vi "NtfyLvFpga_SUB_SettingPanel.vi"(8 "Prohibit time":T1, 10 "SendTo":T2, 11 "SMTP Setting":T3={"smtp server"="", "From"="", "port number"=25, "chk smtp auth"=FALSE, "userID"="", "password"="", "chk ssl"=FALSE}) -> (0 "Prohibit time out":T1, 1 "OK?":bool, 2 "SendTo out":T2, 3 "SMTP Setting out":T3={"smtp server"="", "From"="", "port number"=25, "chk smtp auth"=FALSE, "userID"="", "password"="", "chk ssl"=FALSE})   [LabVIEW 2013]
uses:
  <vilib>/Utility/miscctls.llb/LVPointTypeDef.ctl
panel:
  in  "Chk Prohibition":bool
  in  "End hour":u8=6 caption=":00" max=23
  in  "Start hour":u8=23 caption=":00 to" max=23
  in  "from":string caption="from address"
  in  "chk ssl":bool
  in  "chk smtp auth":bool=TRUE
  in  "password":string
  in  "userID":string
  in  "port number":i32=25
  in  "smtp server":string
  in  "To 3":string caption="To: 3"
  in  "chk To 3":bool
  in  "To 2":string="@ezweb.ne.jp" caption="To: 2"
  in  "chk To 2":bool
  in  "To 1":string caption="To: 1 (必須)"
  in  "chk To 1":bool=TRUE
  in  "Btn Test":bool
  in  "Btn Cancel":bool
  in  "Btn OK":bool
  # "Setting"
  # "SMTP Server and Account"
  # "メールサーバ"
  # "送信者メールアドレス"
  # "Notify Mail Send To:"
  # "有効"
  # "Prohibition time of mail send"
  # "の時間帯はメール送信しない。蓄積して後でまとめて送信。"
  # "同じ時刻を指定した場合は無視されます。"
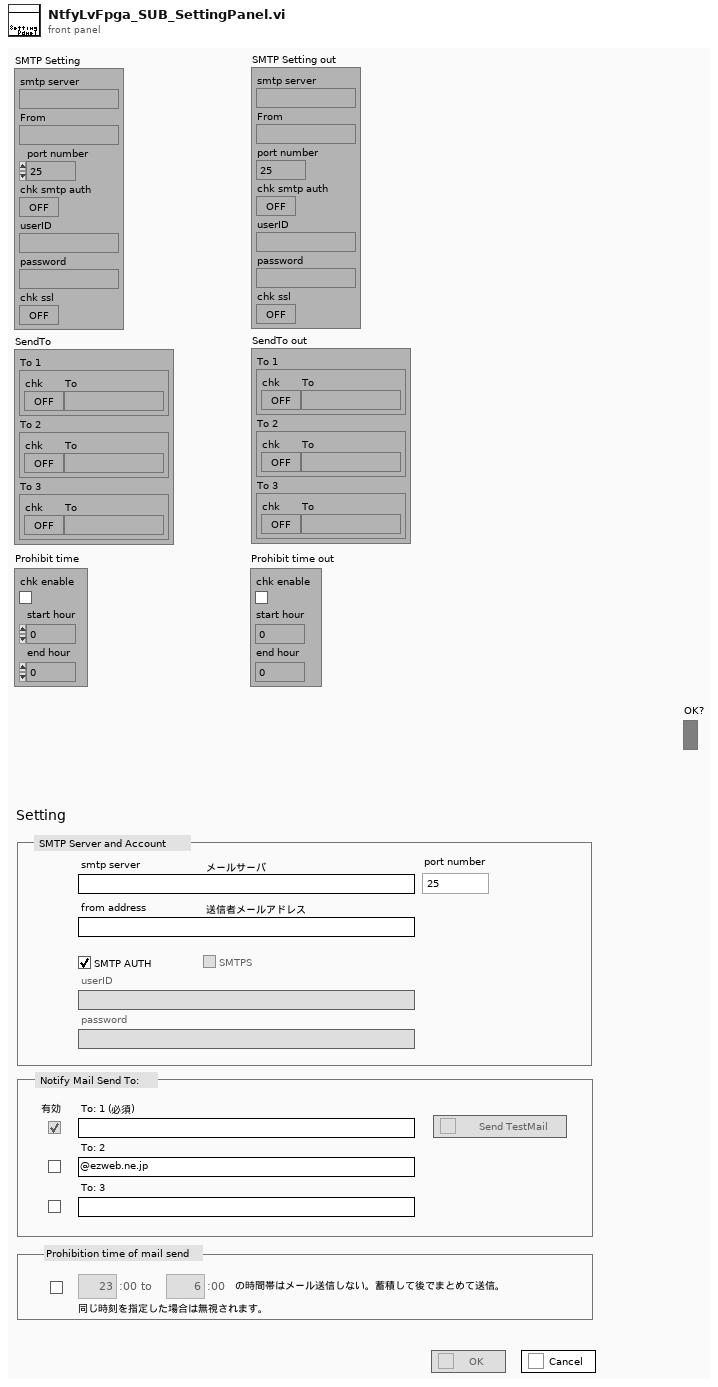
[diagram p1: front panel]
types:
  T1 = cluster{"chk enable":bool, "start hour":u8, "end hour":u8}
  T2 = cluster{"To 1":cluster{"chk":bool, "To":string}, "To 2":cluster{"chk":bool, "To":string}, "To 3":cluster{"chk":bool, "To":string}}
  T3 = cluster{"smtp server":string, "From":string, "port number":i32, "chk smtp auth":bool, "userID":string, "password":string, "chk ssl":bool}
  T4 = typedef "LVPointTypeDef.ctl" = cluster{"Horizontal":i16, "Vertical":i16}
  T5 = enum8{"Enabled", "Disabled", "Disabled and Grayed Out"}
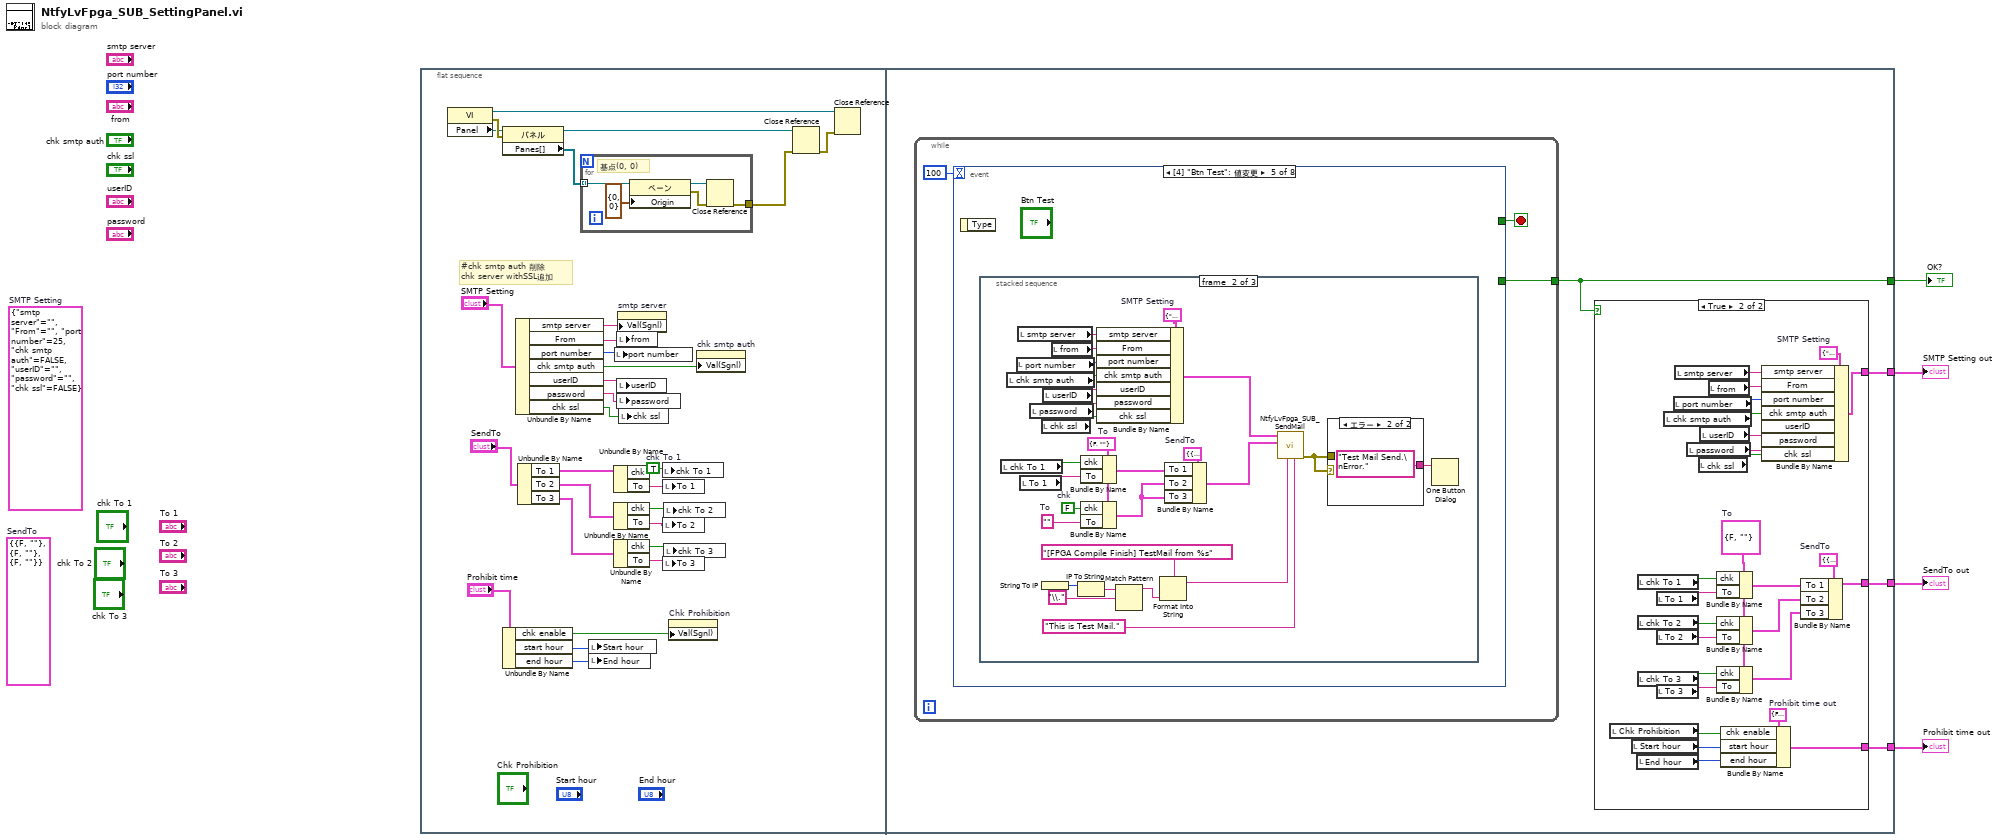
[diagram p0: block diagram]
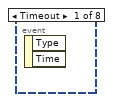
[diagram p3: hidden frame]
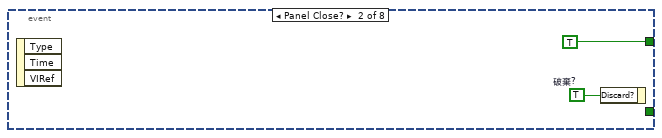
[diagram p4: hidden frame]
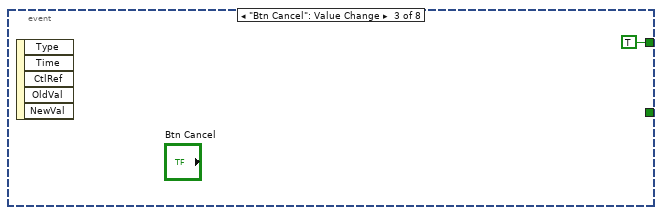
[diagram p5: hidden frame]
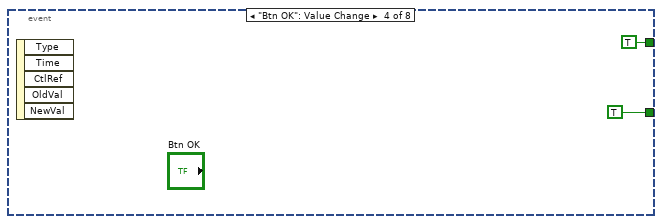
[diagram p6: hidden frame]
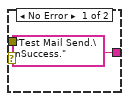
[diagram p8: hidden frame]
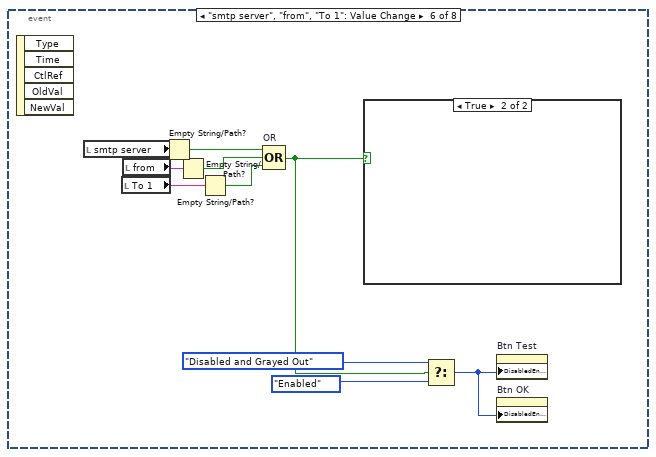
[diagram p10: hidden frame]
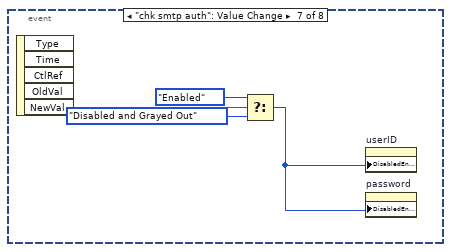
[diagram p12: hidden frame]
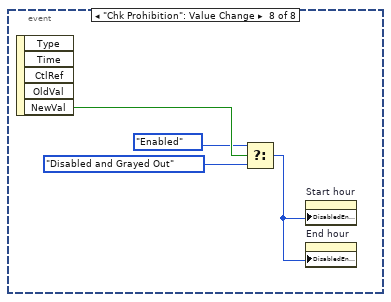
[diagram p13: hidden frame]
diagram:
  (unwired) T2 {"To 1"={"chk"=FALSE, "To"=""}, "To 2"={"chk"=FALSE, "To"=""}, "To 3"={"chk"=FALSE, "To"=""}}  # SendTo
  (unwired) T3 {"smtp server"="", "From"="", "port number"=25, "chk smtp auth"=FALSE, "userID"="", "password"="", "chk ssl"=FALSE}  # SMTP Setting
  n1 = flat-sequence {
    tunnel: [w42] -> w4
    tunnel: [w41] -> w3
    tunnel: [w40] -> w2
    tunnel: [w39] -> w1
    frame #0 {
      w11 = TRUE  # chk To 1
      # "#chk smtp auth 削除\nchk server withSSL追加"
      n2 = property class="VI"() -> (reference out=w30:refnum<vi>, error out=w33:errorcluster, "Panel"=w27:refnum<vi>)  [unwired: 2 in]
      n3 = Unbundle By Name("Prohibit time") -> ("chk enable"=w7:bool, "start hour"=w6:u8, "end hour"=w5:u8)
      n4 = property on="プロパティノード" class="パネル"(reference=w27, error in=w33) -> (reference out=w29:refnum<vi>, "Panes[]"=w28:refnum<vi>[])  [unwired: 1 out]
      n5 = Unbundle By Name("SMTP Setting") -> ("smtp server"=w10:string, "From"=w25:string, "port number"=w24:i32, "chk smtp auth"=w9:bool, "userID"=w23:string, "password"=w22:string, "chk ssl"=w21:bool)
      n6 = Unbundle By Name("SendTo") -> ("To 1"=w19:cluster{"chk":bool, "To":string}, "To 2"=w18:cluster{"chk":bool, "To":string}, "To 3"=w17:cluster{"chk":bool, "To":string})
      n7 = for {
        tunnel: w28 -> [w38] mode=indexing
        tunnel: [w35] -> w31
        # "基点(0, 0)"
        n8 = property on="プロパティノード" class="ペーン"(reference=w38, "Origin"=T4 {"Horizontal"=0, "Vertical"=0} ("原点")) -> (reference out=w37:refnum<vi>, error out=w36:errorcluster)  [unwired: 1 in]
        n9 = Close Reference(reference=w37, error in (no error)=w36) -> (error out=w35:errorcluster)
      }
      n10 = local write "Start hour"(w6) -> ()
      n11 = local write "End hour"(w5) -> ()
      n12 = Unbundle By Name(w19) -> ("To"=w14:string)  [unwired: 1 out]
      n13 = Unbundle By Name(w18) -> ("chk"=w12:bool, "To"=w15:string)
      n14 = Unbundle By Name(w17) -> ("chk"=w13:bool, "To"=w16:string)
      n15 = local write "port number"(w24) -> ()
      n16 = local write "from"(w25) -> ()
      n17 = local write "userID"(w23) -> ()
      n18 = local write "password"(w22) -> ()
      n19 = property on="smtp server" class="Str"("Val(Sgnl)"=w10) -> ()  [unwired: 2 in, 2 out]
      n20 = local write "chk ssl"(w21) -> ()
      n21 = local write "chk To 1"(w11) -> ()
      n22 = local write "To 1"(w14) -> ()
      n23 = local write "To 2"(w15) -> ()
      n24 = local write "To 3"(w16) -> ()
      n25 = local write "chk To 2"(w12) -> ()
      n26 = local write "chk To 3"(w13) -> ()
      n27 = property on="Chk Prohibition" class="Bool （指定）"("Val(Sgnl)"=w7) -> ()  [unwired: 2 in, 2 out]
      n28 = property on="chk smtp auth" class="Bool （指定）"("Val(Sgnl)"=w9) -> ()  [unwired: 2 in, 2 out]
      n29 = Close Reference(reference=w29, error in (no error)=w31) -> (error out=w32:errorcluster)
      n30 = Close Reference(reference=w30, error in (no error)=w32) -> ()  [unwired: 1 out]
    }
    frame #1 {
      n31 = while {
        tunnel: [w69] -> w42
        stop <- w70 stop-if-true
        n32 = event shown="[4] \"Btn Test\": 値変更" {
          selector: _ -> [_ _ _ _ _ _ _ _]
          dyn-events: _ -> [_ _ _ _ _ _ _ _]
          timeout: 100 -> [_ _ _ _ _ _ _ _]
          tunnel: [_ TRUE TRUE TRUE _ _ _ _] -> w70
          tunnel: [_ _ _ TRUE _ _ _ _] -> w69
          event Timeout {
            n33 = event-data() -> ()  [unwired: 1 in, 2 out]
          }
          event Panel Close? {
            w73 = TRUE  # 破棄?
            n34 = event-data() -> ()  [unwired: 1 in, 3 out]
            n35 = event-data("Discard?"=w73) -> ()  [unwired: 1 in, 1 out]
          }
          event "Btn Cancel": Value Change {
            n36 = event-data() -> ()  [unwired: 1 in, 5 out]
          }
          event "Btn OK": Value Change {
            n37 = event-data() -> ()  [unwired: 1 in, 5 out]
          }
          event "Btn Test": Value Change {
            n38 = event-data() -> ()  [unwired: 1 in, 1 out]
            n39 = stacked-sequence {
              frame #0 {
              }
              frame #1 {
                w95 = ""  # To
                w88 = FALSE  # chk
                w92 = cluster{"chk":bool, "To":string} {"chk"=FALSE, "To"=""}  # To
                w93 = T2 {"To 1"={"chk"=FALSE, "To"=""}, "To 2"={"chk"=FALSE, "To"=""}, "To 3"={"chk"=FALSE, "To"=""}}  # SendTo
                w96 = T3 {"smtp server"="", "From"="", "port number"=25, "chk smtp auth"=FALSE, "userID"="", "password"="", "chk ssl"=FALSE}  # SMTP Setting
                n40 = local read "chk To 1"() -> (w90:bool)
                n41 = local read "chk smtp auth"() -> (w84:bool)
                n42 = local read "port number"() -> (w98:i32)
                n43 = local read "smtp server"() -> (w100:string)
                n44 = local read "To 1"() -> (w89:string)
                n45 = local read "password"() -> (w86:string)
                n46 = local read "chk ssl"() -> (w97:bool)
                n47 = String To IP() -> (0:w80:u32)  [unwired: 1 in]
                n48 = local read "userID"() -> (w85:string)
                n49 = local read "from"() -> (w99:string)
                n50 = IP To String(2:w80) -> (0:w79:string)  [unwired: 1 in]
                n51 = Bundle By Name(cluster=w92, "chk"=w90, "To"=w89) -> (w91:cluster{"chk":bool, "To":string})
                n52 = Bundle By Name(cluster=w92, "chk"=w88, "To"=w95) -> (w94:cluster{"chk":bool, "To":string})
                n53 = Bundle By Name(cluster=w96, "smtp server"=w100, "From"=w99, "port number"=w98, "chk smtp auth"=w84, "userID"=w85, "password"=w86, "chk ssl"=w97) -> (w83:T3)
                n54 = Match Pattern(string=w79, regular expression="\\.") -> (before substring=w77:string)  [unwired: 1 in, 3 out]
                n55 = Format Into String(format string="[FPGA Compile Finish] TestMail from %s", w77) -> (resulting string=w81:string)  [unwired: 2 in, 1 out]
                n56 = Bundle By Name(cluster=w93, "To 1"=w91, "To 2"=w94, "To 3"=w94) -> (w87:T2)
                n57 = call "NtfyLvFpga_SUB_SendMail.vi"("Body"="This is Test Mail.", "Subject"=w81, "SendTo"=w87, "SMTP Setting"=w83) -> ("error out"=w102:errorcluster)  [unwired: 7 in]
                n58 = case shown="エラー" w102 {
                  tunnel: w102 -> [_ _]
                  tunnel: ["Test Mail Send.\nSuccess." "Test Mail Send.\nError."] -> w103
                  frame No Error {
                  }
                  frame Error {
                  }
                }
                n59 = One Button Dialog(message=w103) -> ()  [unwired: 1 in, 1 out]
              }
              frame #2 {
              }
            }
          }
          event "smtp server", "from", "To 1": Value Change {
            n60 = event-data() -> ()  [unwired: 1 in, 5 out]
            n61 = local read "smtp server"() -> (w115:string)
            n62 = local read "To 1"() -> (w113:string)
            n63 = local read "from"() -> (w114:string)
            n64 = Empty String/Path?(string/path=w115) -> (empty?=w112:bool)
            n65 = Empty String/Path?(string/path=w114) -> (empty?=w111:bool)
            n66 = Empty String/Path?(string/path=w113) -> (empty?=w110:bool)
            n67 = Compound Arithmetic op=OR "OR"(w112, w111, w110) -> (w107:bool)
            n68 = case shown="TRUE" w107 {
              frame False {
              }
              frame True {
              }
            }
            n69 = Select(t=T5."Disabled and Grayed Out", s=w107, f=T5."Enabled") -> (s? t:f=w106:T5)
            n70 = property on="Btn Test" class="Bool"("DisabledEnum"=w106) -> ()  [unwired: 2 in, 2 out]
            n71 = property on="Btn OK" class="Bool"("DisabledEnum"=w106) -> ()  [unwired: 2 in, 2 out]
          }
          event "chk smtp auth": Value Change {
            n72 = event-data() -> ("NewVal"=w119:bool)  [unwired: 1 in, 4 out]
            n73 = Select(t=T5."Enabled", s=w119, f=T5."Disabled and Grayed Out") -> (s? t:f=w116:T5)
            n74 = property on="userID" class="Str"("DisabledEnum"=w116) -> ()  [unwired: 2 in, 2 out]
            n75 = property on="password" class="Str"("DisabledEnum"=w116) -> ()  [unwired: 2 in, 2 out]
          }
          event "Chk Prohibition": Value Change {
            n76 = event-data() -> ("NewVal"=w123:bool)  [unwired: 1 in, 4 out]
            n77 = Select(t=T5."Enabled", s=w123, f=T5."Disabled and Grayed Out") -> (s? t:f=w120:T5)
            n78 = property on="Start hour" class="DigNum （指定）"("DisabledEnum"=w120) -> ()  [unwired: 2 in, 2 out]
            n79 = property on="End hour" class="DigNum （指定）"("DisabledEnum"=w120) -> ()  [unwired: 2 in, 2 out]
          }
        }
      }
      n80 = case shown="TRUE" w42 {
        tunnel: [_ w67] -> w41
        tunnel: [_ w65] -> w40
        tunnel: [_ w43] -> w39
        frame False {
        }
        frame True {
          w47 = T1 {"chk enable"=FALSE, "start hour"=0, "end hour"=0}  # Prohibit time out
          w57 = cluster{"chk":bool, "To":string} {"chk"=FALSE, "To"=""}  # To
          w66 = T2 {"To 1"={"chk"=FALSE, "To"=""}, "To 2"={"chk"=FALSE, "To"=""}, "To 3"={"chk"=FALSE, "To"=""}}  # SendTo
          w68 = T3 {"smtp server"="", "From"="", "port number"=25, "chk smtp auth"=FALSE, "userID"="", "password"="", "chk ssl"=FALSE}  # SMTP Setting
          n81 = local read "Chk Prohibition"() -> (w46:bool)
          n82 = local read "Start hour"() -> (w45:u8)
          n83 = local read "End hour"() -> (w44:u8)
          n84 = local read "chk To 1"() -> (w53:bool)
          n85 = local read "chk To 2"() -> (w51:bool)
          n86 = local read "chk To 3"() -> (w49:bool)
          n87 = local read "To 1"() -> (w52:string)
          n88 = local read "To 2"() -> (w50:string)
          n89 = local read "To 3"() -> (w48:string)
          n90 = local read "chk smtp auth"() -> (w61:bool)
          n91 = local read "port number"() -> (w58:i32)
          n92 = local read "smtp server"() -> (w60:string)
          n93 = local read "password"() -> (w63:string)
          n94 = local read "chk ssl"() -> (w64:bool)
          n95 = local read "userID"() -> (w62:string)
          n96 = local read "from"() -> (w59:string)
          n97 = Bundle By Name(cluster=w57, "chk"=w53, "To"=w52) -> (w56:cluster{"chk":bool, "To":string})
          n98 = Bundle By Name(cluster=w57, "chk"=w51, "To"=w50) -> (w55:cluster{"chk":bool, "To":string})
          n99 = Bundle By Name(cluster=w55, "chk"=w49, "To"=w48) -> (w54:cluster{"chk":bool, "To":string})
          n100 = Bundle By Name(cluster=w47, "chk enable"=w46, "start hour"=w45, "end hour"=w44) -> (w43:T1)
          n101 = Bundle By Name(cluster=w68, "smtp server"=w60, "From"=w59, "port number"=w58, "chk smtp auth"=w61, "userID"=w62, "password"=w63, "chk ssl"=w64) -> (w67:T3)
          n102 = Bundle By Name(cluster=w66, "To 1"=w56, "To 2"=w55, "To 3"=w54) -> (w65:T2)
        }
      }
    }
  }
  "OK?" <- w4
  "SendTo out" <- w2
  "SMTP Setting out" <- w3
  "Prohibit time out" <- w1
